vi "DrawLandmarks.vi"(8 "error in (no error)":errorcluster, 10 "Landmarks":cluster{"X position":dbl, "Y position":dbl}[](array[cluster]), 11 "picture":picture) -> (0 "error out":errorcluster, 3 "new picture":picture)   [LabVIEW 2009, in "Host.lvlib" / "Draw.lvlib"]
uses:
  Draw.lvlib
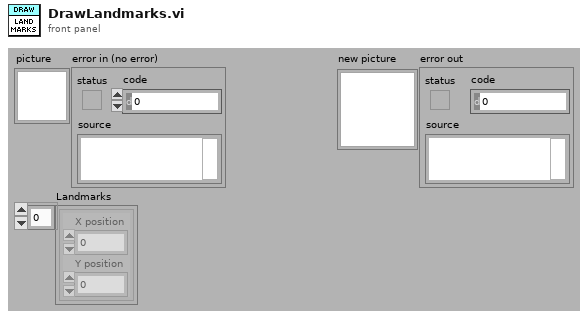
[diagram p1: front panel]
types:
  T1 = cluster{"Width":u16, "Style":enum32{"Solid", "Dash", "Dot", "DashDot", "DashDotDot"}}
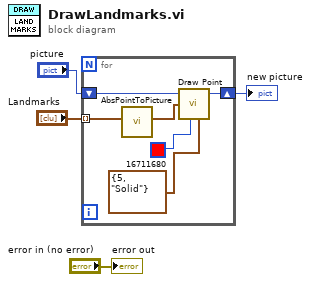
[diagram p0: block diagram]
diagram:
  n1 = for {
    tunnel: "Landmarks" -> [w10] mode=indexing
    shift-right: [w7] -> w2
    shift-left: "picture" -> [w8]
    n2 = call "AbsPointToPicture.vi"("input position"=w10) -> ("output point"=w9:cluster{"x":i16, "y":i16})  [unwired: 10 in]
    n3 = call <vilib>:"Draw Point.vi"("picture"=w8, "point(x,y)"=w9, "color(black)"=u32 16711680, "pen"=T1 {"Width"=5, "Style"=enum."Solid"}) -> ("new picture"=w7:picture)  [unwired: 5 in]
  }
  "new picture" <- w2
  "error out" <- "error in (no error)"
